vi "Untitled 3.vi"() -> ()   [LabVIEW 2017]
panel:
  in  "Boolean":bool
  out "date/time string":string
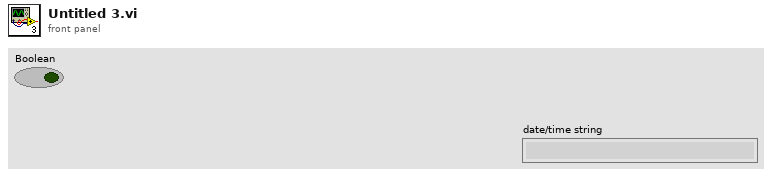
[diagram p1: front panel]
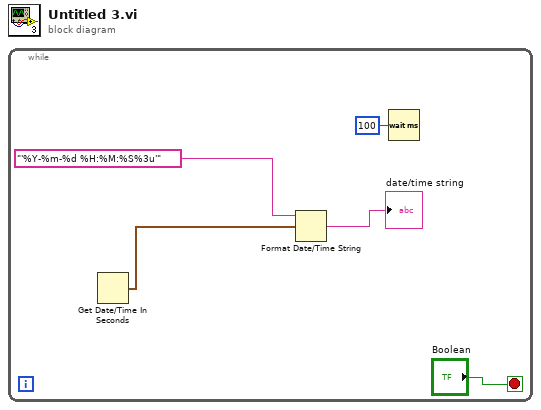
[diagram p0: block diagram]
diagram:
  n1 = while {
    stop <- "Boolean" stop-if-true
    n2 = Get Date/Time In Seconds() -> (seconds since 1Jan1904=w1:timestamp)
    n3 = Format Date/Time String(time format string (%c)="'%Y-%m-%d %H:%M:%S%3u'", seconds (now)=w1) -> (date/time string=→"date/time string":string)  [unwired: 1 in]
    n4 = Wait (ms)(milliseconds to wait=u32 100) -> ()  [unwired: 1 out]
  }
